vi "SDG60ReadParameters.vi"(7 "Timeout (40000 ms)":u32=40000, 8 "error in (no error)":errorcluster, 9 "Function Type (0: Basic)":u16(ring) items=["Basic Wave", "Modulate Wave ", "Sweep Wave", "Burst Wave", "Sample Rate"], 10 "Channel (1:Channel 1)":i32(ring)=1 items=["Channel 1"=1, "Channel 2"=2], 11 "VISA resource name":refnum<visa-resource-name>="USB0::0xF4EC::0x1101::SDG6XEBC5R0119::INSTR") -> (0 "error out":errorcluster, 2 "String":string, 3 "VISA resource name out":refnum<visa-resource-name>)   [LabVIEW 2018]
doc: "Creates and saves an arbitrary waveform in edit memory. \n\n<B>Note:</B>\n\nCreates an arbitrary waveform in edit memory and because of this, the waveform will remain stored on the instrument until deleted. If any sensitive information is contained in the arbitrary waveform, it is recommended that the waveform be deleted when finished."
panel:
  # "Basic will read user made Arb functions too, but will read freq not sample rate\nuse sample rate function type to read this."
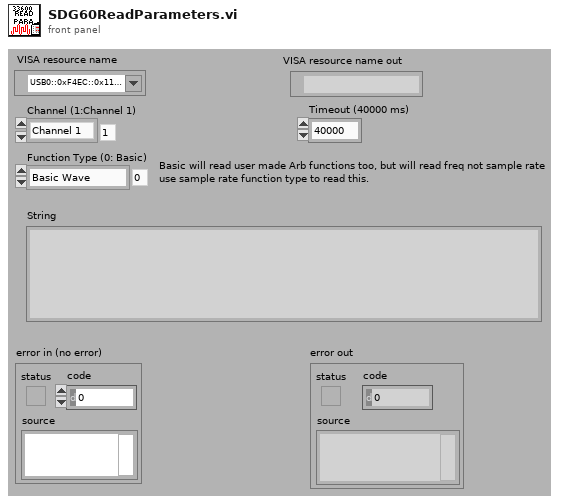
[diagram p1: front panel]
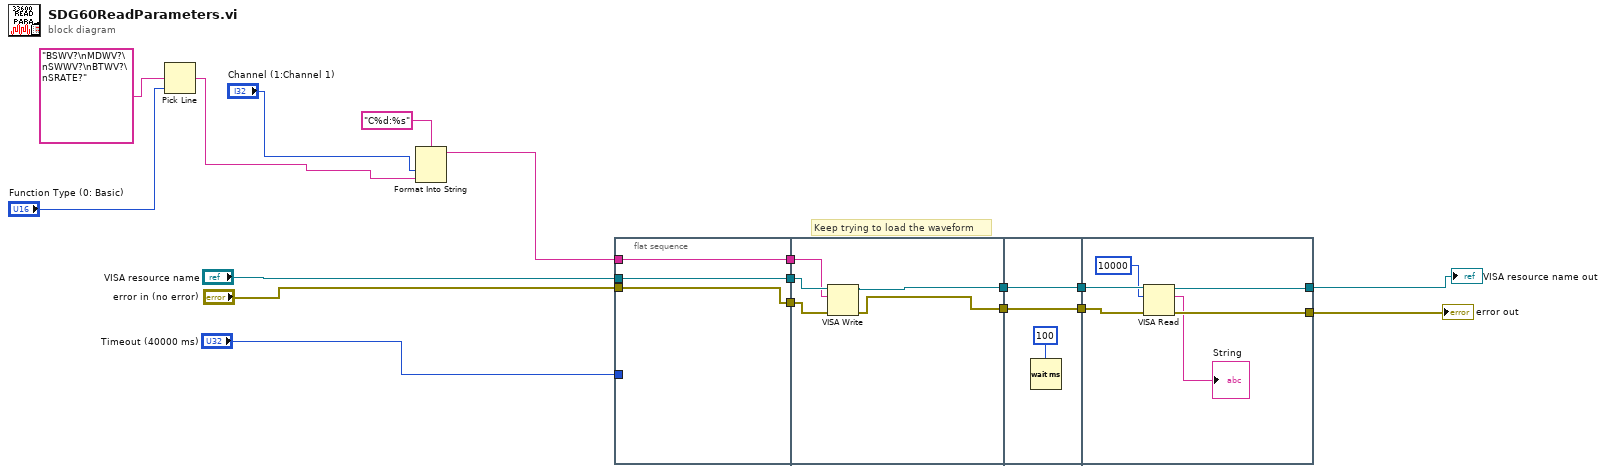
[diagram p0: block diagram]
diagram:
  # "Keep trying to load the waveform"
  n1 = Pick Line(multi-line string="BSWV?\nMDWV?\nSWWV?\nBTWV?\nSRATE?", line index="Function Type (0: Basic)") -> (output string=w2:string)  [unwired: 1 in]
  n2 = Format Into String(format string="C%d:%s", "Channel (1:Channel 1)", w2) -> (resulting string=w13:string)  [unwired: 2 in, 1 out]
  n3 = flat-sequence {
    tunnel: [w19] -> w12
    tunnel: [w20] -> w11
    tunnel: w13 -> [w21]
    tunnel: [w21] -> w10
    tunnel: "Timeout (40000 ms)" -> [_]
    tunnel: "VISA resource name" -> [w19]
    tunnel: "error in (no error)" -> [w20]
    tunnel: w12 -> [w25]
    tunnel: w11 -> [w26]
    tunnel: w10 -> [w24]
    tunnel: [w22] -> w9
    tunnel: [w23] -> w8
    tunnel: w9 -> [w29]
    tunnel: [w29] -> w7
    tunnel: w8 -> [w28]
    tunnel: [w28] -> w6
    tunnel: [w34] -> w15
    tunnel: w7 -> [w33]
    tunnel: w6 -> [w35]
    tunnel: [w32] -> w5
    frame #0 {
    }
    frame #1 {
      n4 = VISA Write(VISA resource name=w25, write buffer=w24, error in (no error)=w26) -> (VISA resource name out=w23:refnum<visa-resource-name>, error out=w22:errorcluster)  [unwired: 1 out]
    }
    frame #2 {
      n5 = Wait (ms)(milliseconds to wait=100 ("x")) -> ()  [unwired: 1 out]
    }
    frame #3 {
      n6 = VISA Read(VISA resource name=w35, byte count=10000 ("x"), error in (no error)=w33) -> (VISA resource name out=w34:refnum<visa-resource-name>, read buffer=→"String":string, error out=w32:errorcluster)  [unwired: 1 out]
    }
  }
  "error out" <- w5
  "VISA resource name out" <- w15
